vi "MDF_Set_Default_Install.vi"(8 "error in (no error)":errorcluster, 11 "IB_Destination in":refnum<class "IB_Destination.lvclass">) -> (0 "error out":errorcluster)   [LabVIEW 2020, in "IB_Destination.lvclass"]
uses:
  <vilib>/AppBuilder/IB_Classes/Destination/IB_Destination.lvclass
  <vilib>/AppBuilder/IB_Classes/Destination/IB_Destination.lvclass/IB_Destination.ctl
  AppLibs/distkit/MDF/NIMdf.llb/MDFBDPAddFilePathType.ctl
  AppLibs/distkit/MDF/NI_MDF.lvlib
  AppLibs/distkit/MDF/NIMdf.llb/MDFBuildDevPart_SetDefaultInstallDir (string).vi
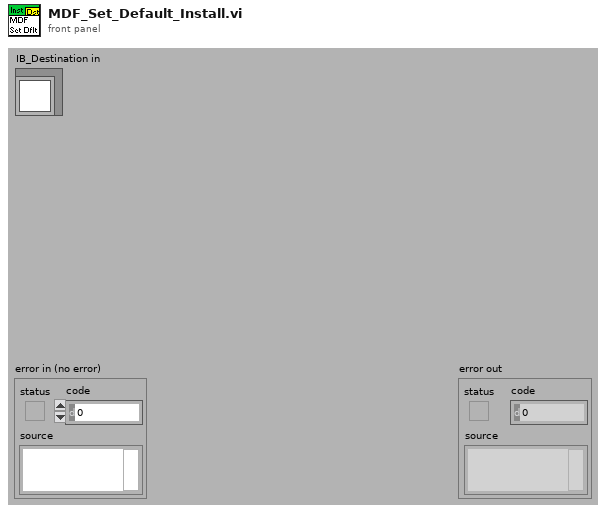
[diagram p1: front panel]
types:
  T1 = typedef "NI_MDF.lvlib/MDFBDPAddFilePathType.ctl" = i32
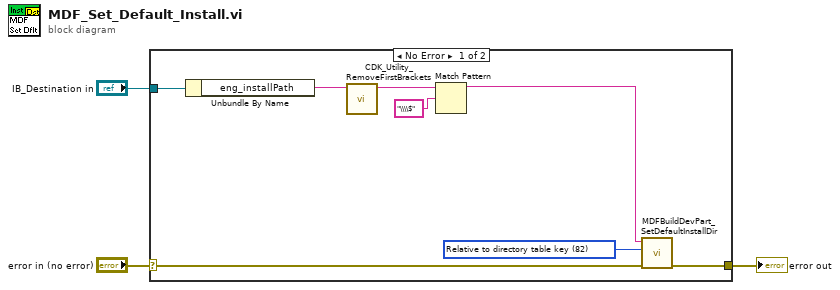
[diagram p0: block diagram]
diagram:
  n1 = case shown="No Error" "error in (no error)" {
    selector: "error in (no error)" -> [w8 w12]
    tunnel: [w7 w12] -> w2
    tunnel: "IB_Destination in" -> [w10 _]
    frame No Error {
      w11 = T1 82 items=["Relative to default installation directory"=68, "Root directory on first partition"=70, "Relative to directory table key"=82, "Absolute path to file"=65] ("installation directory path type (Root directory on first partition)")
      n2 = Unbundle By Name(w10) -> ("eng_installPath"=w9:string)
      n3 = call <resource>:"CDK_Utility_RemoveFirstBrackets.vi"("StringIn"=w9) -> ("StringOut"=w5:string)  [unwired: 1 in, 9 out]
      n4 = Match Pattern(string=w5, regular expression="\\\\$") -> (before substring=w4:string)  [unwired: 1 in, 3 out]
      n5 = call-poly "MDFBuildDevPart_SetDefaultInstallDir.vi"("error in (no error)"=w8, "installation directory path type (Root directory on first partition)"=w11, "default installation directory"=w4) -> ("error out"=w7:errorcluster)  [unwired: 8 in]
    }
    frame Error {
    }
  }
  "error out" <- w2
